vi "Configure Analog Gen References.vi"(6 "Watt Impedance Reference (8 Ohms)":dbl=8.0, 7 "Decibel Relative Reference (1 Vrms)":dbl=1.0, 8 "error in (no error)":errorcluster, 9 "Decibel Impendance Reference (600 ohms)":dbl=600.0, 10 "Frequency Reference (1000 Hz)":dbl=1000.0, 11 "VISA resource name":refnum<visa-resource-name>) -> (0 "error out":errorcluster, 3 "VISA resource name out":refnum<visa-resource-name>)   [LabVIEW 2014, in "Stanford Research SR1.lvlib"]
doc: "Configures the attributes for the Analog Generator References."
uses:
  Stanford Research SR1.lvlib
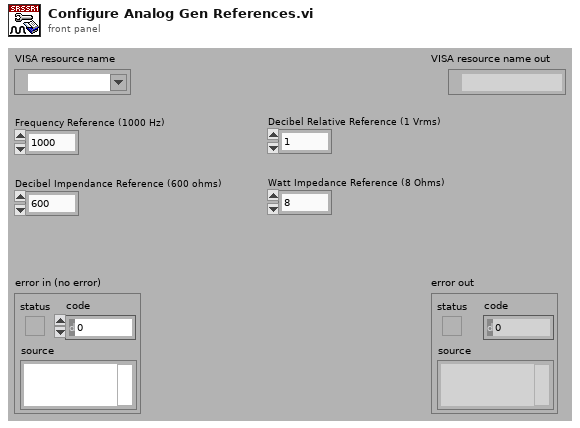
[diagram p1: front panel]
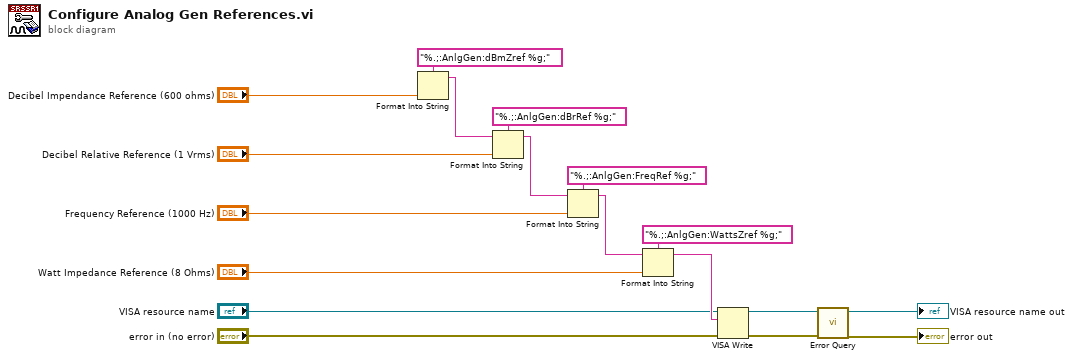
[diagram p0: block diagram]
diagram:
  n1 = Format Into String(format string="%.;:AnlgGen:dBmZref %g;", "Decibel Impendance Reference (600 ohms)") -> (resulting string=w16:string)  [unwired: 2 in, 1 out]
  n2 = Format Into String(format string="%.;:AnlgGen:dBrRef %g;", initial string=w16, "Decibel Relative Reference (1 Vrms)") -> (resulting string=w13:string)  [unwired: 1 in, 1 out]
  n3 = Format Into String(format string="%.;:AnlgGen:FreqRef %g;", initial string=w13, "Frequency Reference (1000 Hz)") -> (resulting string=w10:string)  [unwired: 1 in, 1 out]
  n4 = Format Into String(format string="%.;:AnlgGen:WattsZref %g;", initial string=w10, "Watt Impedance Reference (8 Ohms)") -> (resulting string=w7:string)  [unwired: 1 in, 1 out]
  n5 = VISA Write(VISA resource name="VISA resource name", write buffer=w7, error in (no error)="error in (no error)") -> (VISA resource name out=w4:refnum<visa-resource-name>, error out=w3:errorcluster)  [unwired: 1 out]
  n6 = call "Error Query.vi"("error in (no error)"=w3, "VISA resource name"=w4) -> ("error out"=→"error out":errorcluster, "VISA resource name out"=→"VISA resource name out":refnum<visa-resource-name>)  [unwired: 6 in, 2 out]
